vi "Working Start Range Waveform.vi"() -> ()   [LabVIEW 2026]
uses:
  <vilib>/numeric/Random Number (Range) U64.vi
  <vilib>/numeric/sub_Random U32.vi
panel:
  in  "Channel Gain (dB)":dbl
  out "Slide":dbl(slide) scale=0.0..10.0
  in  "Range":dbl
  in  "Start":dbl
  out "Channel 1":u64[](graph)
  # "zeT9EBE&Y%.?2gk"
  # "A-Scan Window"
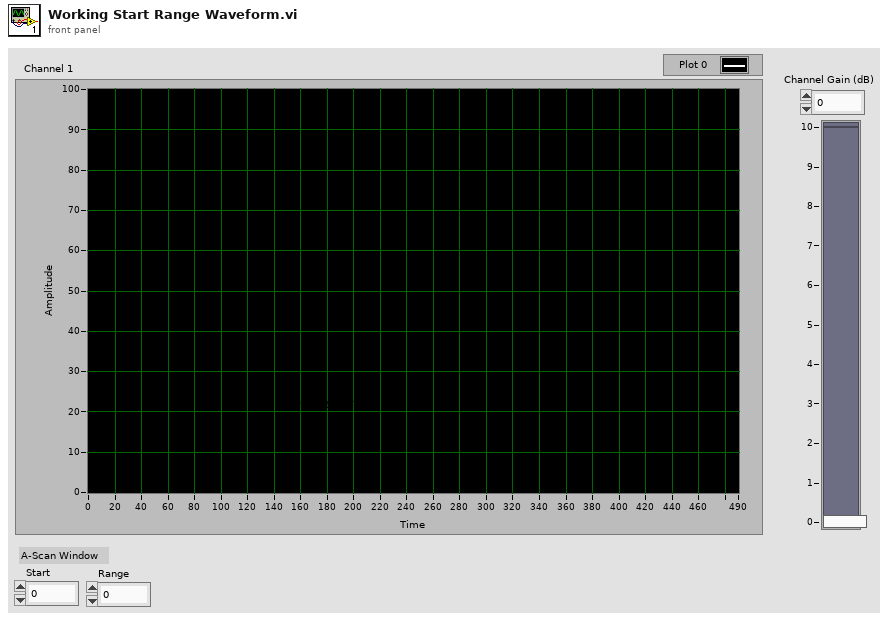
[diagram p1: front panel]
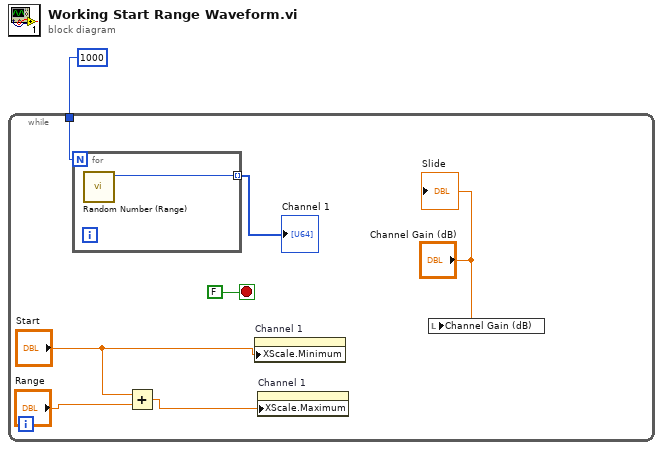
[diagram p0: block diagram]
diagram:
  n1 = while {
    tunnel: 1000 -> [w8]
    stop <- FALSE stop-if-true
    n2 = for {
      N: w8 -> [_]
      tunnel: [w9] -> w6 mode=indexing
      n3 = call-poly <vilib>:"Random Number (Range).vi"() -> ("number"=w9:u64)  [unwired: 11 in]
    }
    "Channel 1" <- w6
    n4 = Add(x="Start", y="Range") -> (x+y=w5:dbl)
    n5 = property on="Channel 1" class="WFGraph (strict)"("XScale.Minimum"="Start") -> ()  [unwired: 2 in, 2 out]
    n6 = property on="Channel 1" class="WFGraph (strict)"("XScale.Maximum"=w5) -> ()  [unwired: 2 in, 2 out]
    n7 = local write "Channel Gain (dB)"("Channel Gain (dB)") -> ()
    "Slide" <- "Channel Gain (dB)"
  }
